vi "SendResult.vi"(7 "result":i32(ring)=2 items=["user and pass no exist", "no match with timeslot", "user ok"], 8 "error in (no error)":errorcluster, 9 "endtime in":string, 10 "starttime in":string, 11 "connection ID in":refnum<k5>) -> (0 "error out":errorcluster, 3 "connection ID out":refnum<k5>)   [LabVIEW 2010]
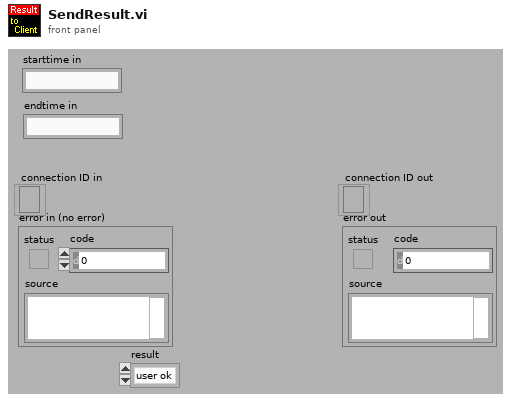
[diagram p1: front panel]
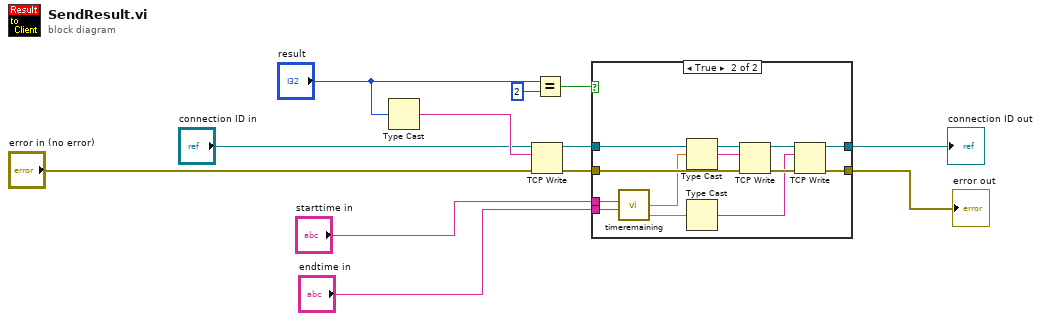
[diagram p0: block diagram]
diagram:
  n1 = Type Cast(x="result") -> (*(type *) &x=w12:string)  [unwired: 1 out]
  n2 = TCP Write(connection ID="connection ID in", data in=w12, error in (no error)="error in (no error)") -> (connection ID out=w9:refnum<k5>, error out=w8:errorcluster)  [unwired: 2 out]
  n3 = Equal?(x="result", y=2) -> (x = y?=w10:bool)
  n4 = case shown="True" w10 {
    tunnel: "starttime in" -> [_ w26]
    tunnel: "endtime in" -> [_ w25]
    tunnel: w9 -> [w14 w24]
    tunnel: w8 -> [w13 w23]
    tunnel: [w14 w20] -> w2
    tunnel: [w13 w19] -> w1
    frame False {
    }
    frame True {
      n5 = call "timeremaining.vi"("endtime"=w25, "starttime"=w26) -> ("time remaining"=w16:sgl, "slot time"=w18:sgl)  [unwired: 3 out]
      n6 = Type Cast(x=w18) -> (*(type *) &x=w17:string)  [unwired: 1 out]
      n7 = Type Cast(x=w16) -> (*(type *) &x=w15:string)  [unwired: 1 out]
      n8 = TCP Write(connection ID=w24, data in=w17, error in (no error)=w23) -> (connection ID out=w21:refnum<k5>, error out=w22:errorcluster)  [unwired: 2 out]
      n9 = TCP Write(connection ID=w21, data in=w15, error in (no error)=w22) -> (connection ID out=w20:refnum<k5>, error out=w19:errorcluster)  [unwired: 2 out]
    }
  }
  "connection ID out" <- w2
  "error out" <- w1
